vi "Wristband char to data.vi"(8 "Error In":errorcluster, 10 "Wristband char value":u8[](array[numeric])) -> (0 "Error Out":errorcluster, 1 "YPR data":cluster{"Yaw":sgl, "Pitch":sgl, "Roll":sgl}, 2 "Strain data":T1)   [LabVIEW 2016]
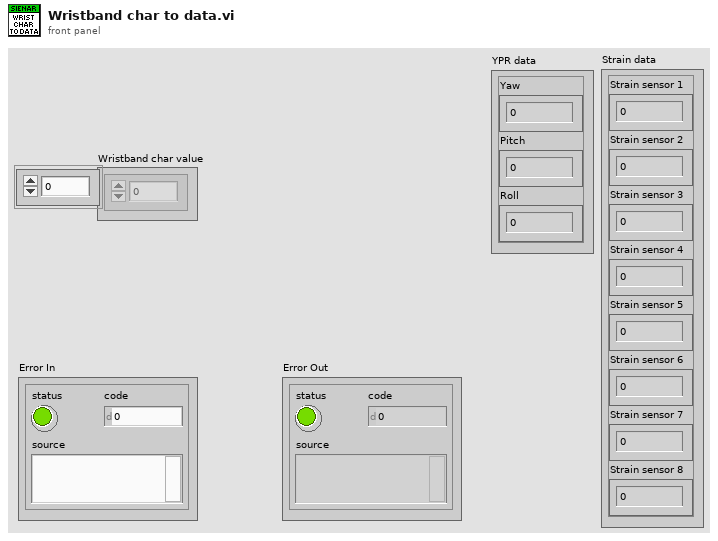
[diagram p1: front panel]
types:
  T1 = cluster{"Strain sensor 1":sgl, "Strain sensor 2":sgl, "Strain sensor 3":sgl, "Strain sensor 4":sgl, "Strain sensor 5":sgl, "Strain sensor 6":sgl, "Strain sensor 7":sgl, "Strain sensor 8":sgl}
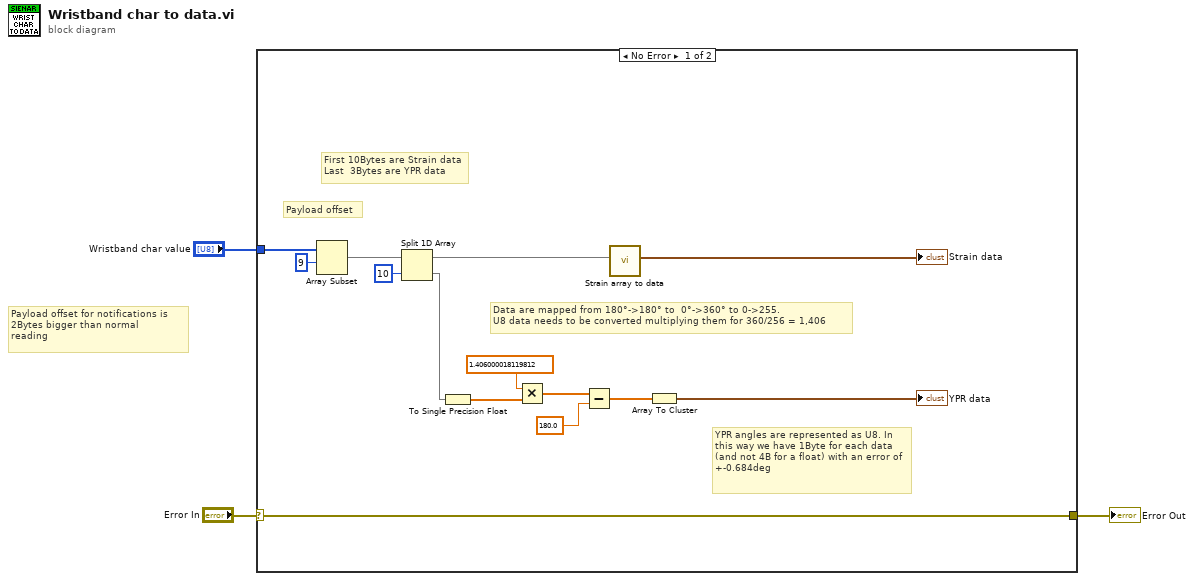
[diagram p0: block diagram]
diagram:
  # "Payload offset for notifications is \n2Bytes bigger than normal\nreading"
  n1 = case shown="No Error" "Error In" {
    selector: "Error In" -> [w17 w18]
    tunnel: [w17 w18] -> w2
    tunnel: "Wristband char value" -> [w15 _]
    frame No Error {
      # "Data are mapped from 180°->180° to  0°->360° to 0->255.\nU8 data needs to be converted multiplying them for 360/256 = 1,406"
      # "YPR angles are represented as U8. In this way we have 1Byte for each data (and not 4B for a float) with an error of +-0.684deg"
      # "First 10Bytes are Strain data\nLast  3Bytes are YPR data"
      # "Payload offset"
      n2 = Array Subset(array=w15, index=9) -> (w14:u8[])  [unwired: 1 in]
      n3 = Split 1D Array(array=w14, index=10) -> (first subarray=w12:u8[], second subarray=w9:u8[])
      n4 = To Single Precision Float(number=w9) -> (single precision float=w11:sgl[])
      n5 = Multiply(x=sgl 1.406, y=w11) -> (x*y=w7:sgl[])
      n6 = Subtract(x=w7, y=sgl 180.0) -> (x-y=w5:sgl[])
      n7 = call "Strain array to data.vi"("Strain array"=w12) -> ("Strain data"=→"Strain data":T1)  [unwired: 9 in, 1 out]
      n8 = Array To Cluster(array=w5) -> (cluster=→"YPR data":cluster{"[0]":sgl, "[1]":sgl, "[2]":sgl})
    }
    frame Error {
    }
  }
  "Error Out" <- w2
